vi "Pipe Var Intf - Write Dbl Matrix.vi"(8 "error in (no error)":errorcluster, 9 "data":dbl[][](array[numeric]), 10 "variable name":string, 11 "GOLPI ref. in":T1={"pipe handle"={"lv_proc.dll file path"=path "", "process instance handle"=[], "debug mode"=FALSE, "debug data"=[]}, "fast read timeout [ms]"=500, "fast read settle time [ms]"=10, "fast read to multiple [ms]"=1, "max elements per input line"=100, "slow read timeout [ms]"=5000, "stdin double format specifier"="%_16e", "max elements per stdout output column"=100, "console mode bitstream"=FALSE, "bitstream first read timeout [ms]"=1000, "bitstream read timeout [ms]"=50, "struct transfer possible"=FALSE, "matlab mode"=FALSE, "var pipe write timeout [ms]"=5000, "variable pipe mode"=FALSE, "variable pipe buffer size [Bytes]"=10000000, "variable pipe block size [Bytes]"=1000000} {"variable pipe block size [Bytes]" format="%.0p"; "variable pipe buffer size [Bytes]" format="%.0p"}) -> (0 "error out":errorcluster, 3 "GOLPI ref. out":T1={"pipe handle"={"lv_proc.dll file path"=path "", "process instance handle"=[], "debug mode"=FALSE, "debug data"=[]}, "fast read timeout [ms]"=500, "fast read settle time [ms]"=10, "fast read to multiple [ms]"=1, "max elements per input line"=100, "slow read timeout [ms]"=5000, "stdin double format specifier"="", "max elements per stdout output column"=100, "console mode bitstream"=FALSE, "bitstream first read timeout [ms]"=1000, "bitstream read timeout [ms]"=50, "struct transfer possible"=FALSE, "matlab mode"=FALSE, "var pipe write timeout [ms]"=5000, "variable pipe mode"=FALSE, "variable pipe buffer size [Bytes]"=10000000, "variable pipe block size [Bytes]"=1000000} {"variable pipe block size [Bytes]" format="%.0p"; "variable pipe buffer size [Bytes]" format="%.0p"})   [LabVIEW 2020, in "GOLPI library.lvlib"]
doc: "Write matrix to Octave using pipe variable interface."
uses:
  GOLPI library.lvlib
  Public/GOLPI reference Type Def.ctl
  LV Process source distribution/Pipe Handle.ctl
  Pipe Var Intf - Data Type.ctl
  LV Process source distribution/LV Process library.lvlib
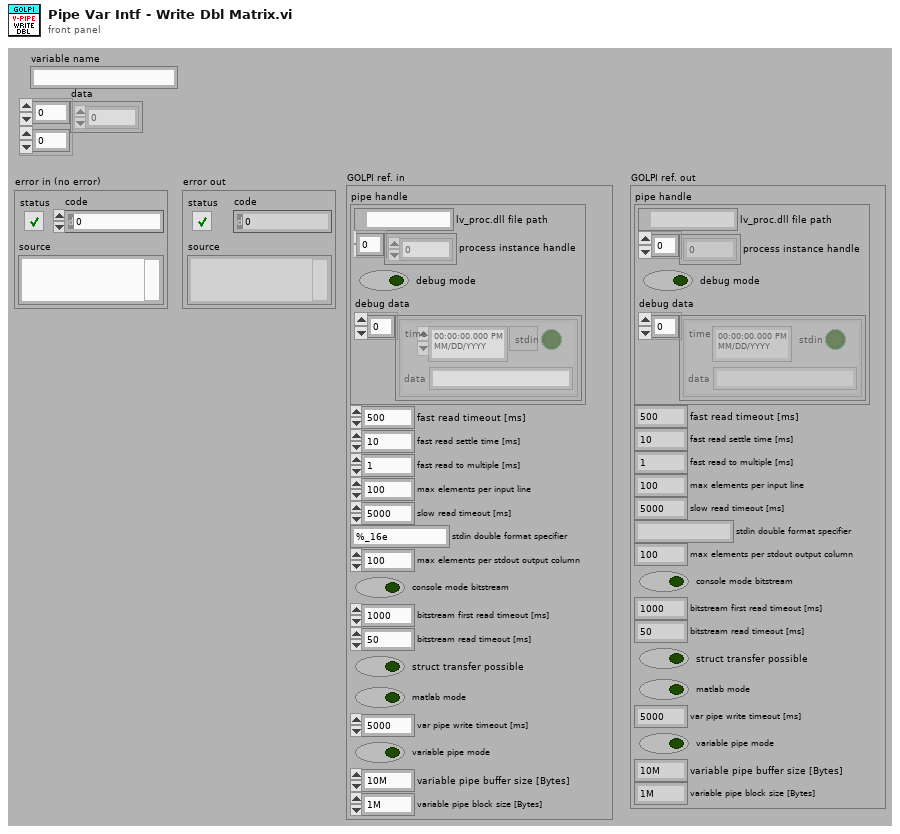
[diagram p1: front panel]
types:
  T1 = typedef "GOLPI library.lvlib/GOLPI reference Type Def.ctl" = cluster{"pipe handle":T2, "fast read timeout [ms]":u32, "fast read settle time [ms]":u32, "fast read to multiple [ms]":u32, "max elements per input line":u32, "slow read timeout [ms]":u32, "stdin double format specifier":string, "max elements per stdout output column":u32, "console mode bitstream":bool, "bitstream first read timeout [ms]":u32, "bitstream read timeout [ms]":u32, "struct transfer possible":bool, "matlab mode":bool, "var pipe write timeout [ms]":u32, "variable pipe mode":bool, "variable pipe buffer size [Bytes]":u32, "variable pipe block size [Bytes]":u32}
  T2 = typedef "LV Process library.lvlib/Pipe Handle.ctl" = cluster{"lv_proc.dll file path":path, "process instance handle":u32[], "debug mode":bool, "debug data":cluster{"time":timestamp, "stdin":bool, "data":string}[]}
  T3 = typedef "GOLPI library.lvlib/Pipe Var Intf - Data Type.ctl" = enum16{"String", "int32", "uint32", "double", "cplx double", "single", "cplx single"}
  T4 = enum16{"big-endian, network order", "native, host order", "little-endian"}
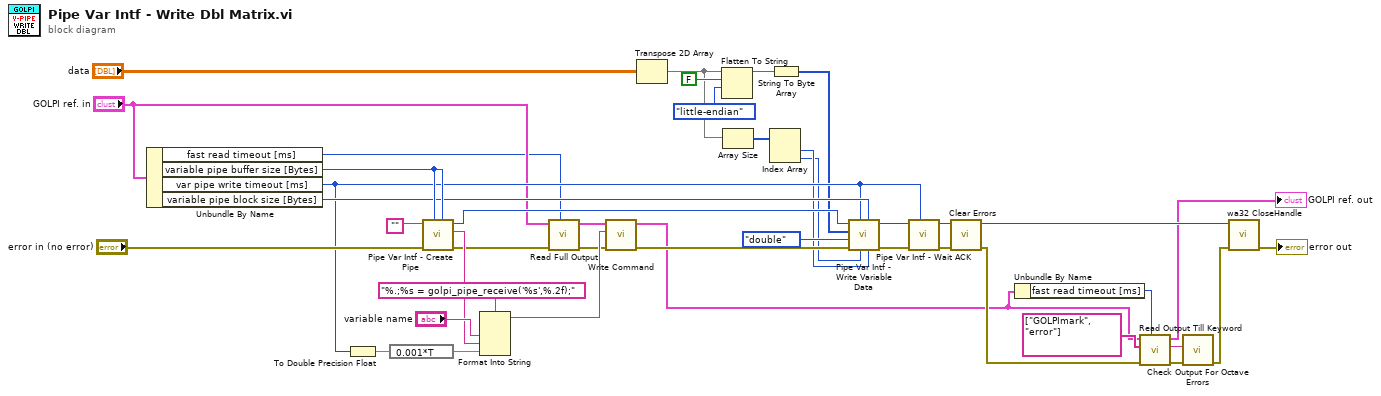
[diagram p0: block diagram]
diagram:
  n1 = Unbundle By Name("GOLPI ref. in") -> ("fast read timeout [ms]"=w4:u32, "variable pipe buffer size [Bytes]"=w26:u32, "var pipe write timeout [ms]"=w23:u32, "variable pipe block size [Bytes]"=w25:u32)
  n2 = To Double Precision Float(number=w23) -> (double precision float=w22:dbl)
  n3 = expression code="0.001*T"(w22) -> (w24:dbl)
  n4 = call "Pipe Var Intf - Create Pipe.vi"("outBufferSize (256k)"=w26, "inBufferSize (256k)"=w26, "error in (no error)"="error in (no error)", "pipe name in (leave empty to generate random name)"="") -> ("error out"=w7:errorcluster, "pipe name out"=w37:string, "pipe handle out"=w35:i32)  [unwired: 5 in]
  n5 = Format Into String(format string="%.;%s = golpi_pipe_receive('%s',%.2f);", "variable name", w37, w24) -> (resulting string=w36:string)  [unwired: 2 in, 1 out]
  n6 = call "Read Full Output.vi"("timeout [ms]"=w4, "error in"=w7, "GOLPI ref. in"="GOLPI ref. in") -> ("error out"=w8:errorcluster, "GOLPI ref. out"=w5:T1)  [unwired: 5 in, 2 out]
  n7 = call "Write Command.vi"("error in"=w8, "command"=w36, "GOLPI ref. in"=w5) -> ("error out"=w40:errorcluster, "GOLPI ref. out"=w9:T1)  [unwired: 7 in]
  n8 = Transpose 2D Array(2D array="data") -> (transposed array=w14:dbl[][])
  n9 = Flatten To String(anything=w14, prepend array or string size? (T)=FALSE, byte order (0:big-endian, network order)=T4."little-endian") -> (data string=w32:string)  [unwired: 1 in, 2 out]
  n10 = Array Size(array=w14) -> (size(s)=w30:i32[])
  n11 = Index Array(array=w30) -> (element #1=w13:i32, element #2=w12:i32)  [unwired: 2 in]
  n12 = String To Byte Array(string=w32) -> (unsigned byte array=w2:u8[])
  n13 = call "Pipe Var Intf - Write Variable Data.vi"("columns"=w13, "write block size (10k)"=w25, "rows"=w12, "timeout [ms]"=w23, "error in (no error)"=w40, "data type"=Pipe_Var_Intf_-_Data_Type."double", "data"=w2, "pipe handle"=w35) -> ("error out"=w1:errorcluster, "pipe handle out"=w27:i32)  [unwired: 2 in]
  n14 = call "Pipe Var Intf - Wait ACK.vi"("timeout [ms]"=w23, "error in (no error)"=w1, "pipe handle"=w27) -> ("error out"=w19:errorcluster, "pipe handle out"=w28:i32)  [unwired: 7 in]
  n15 = call <vilib>:"Clear Errors.vi"("error in (no error)"=w19) -> ("error out"=w11:errorcluster)  [unwired: 5 in, 1 out]
  n16 = Unbundle By Name(w9) -> ("fast read timeout [ms]"=w20:u32)
  n17 = call "Read Output Till Keyword.vi"("timeout [ms]"=w20, "error in"=w11, "keywords"=string[] ["GOLPImark", "error"], "GOLPI ref. in"=w9) -> ("error out"=w18:errorcluster, "read buffer"=w17:string, "GOLPI ref. out"=→"GOLPI ref. out":T1)  [unwired: 4 in, 1 out]
  n18 = call "Check Output For Octave Errors.vi"("error in"=w18, "read buffer"=w17) -> ("error out"=w10:errorcluster)  [unwired: 9 in]
  n19 = call "wa32 CloseHandle.vi"("error in"=w10, "handle"=w28) -> ("error out"=→"error out":errorcluster)  [unwired: 9 in]
